vi "Numeric Indicator - Ring.vi"() -> ()   [LabVIEW 2013, in "Ring Workspace Object.lvlib"]
doc: "Sample numeric display item."
uses:
  Ring Workspace Object.lvlib
  <vilib>/NI Veristand/Display Template Support/Display Template Support.llb/cluster_Screen Item Settings.ctl
  <vilib>/NI Veristand/Display Template Support/Display Template Support.llb/cluster_Graph Scale Settings.ctl
  <vilib>/NI Veristand/Display Template Support/Display Template Support.llb/cluster_Graph Plot Settings.ctl
  NationalInstruments.VeriStand.SystemStorage
  <vilib>/NI Veristand/Display Template Support/Display Template Support.llb/enum_Display Template Handler Minimal To Widget Msg.ctl
  <vilib>/NI Veristand/Display Template Support/Display Template Support.llb/enum_Display Template Handler Minimal To Workspace.ctl
  Types/Saved State Data.ctl
  <vilib>/NI Veristand/Display Template Support/Display Template Support.llb/sub_Display Template Handler Custom.vi
  <vilib>/NI Veristand/Execution/Workspace/NI VeriStand - Get Single Channel Value.vi
  <vilib>/NI Veristand/Execution/Workspace/NI_VS Workspace ExecutionAPI.lvlib
panel:
  out "Ring":i64(ring) caption="Channel"
  in  "NIVS.System Definition Root":refnum<k24>
  in  "Item.Data":T1
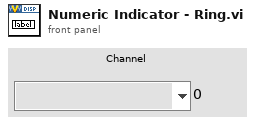
[diagram p1: front panel]
types:
  T1 = typedef "cluster_Screen Item Settings.ctl" = cluster{"Template VI":string, "Position X":i32, "Position Y":i32, "Custom":string, "Show Title Bar":bool, "ID":i32, "Always On Top":bool, "Allow Resize":bool, "Allow Minimize":bool, "Allow Close":bool, "Size to Screen":bool, "Screen.ID":i32, "State":enum16{"Normal", "New"}, "Title":string, "Window Bounds":cluster{"[0]":i16, "[1]":i16, "[2]":i16, "[3]":i16}, "Channel Ref":u64, "Unit":string, "Default Units?":bool, "Flash Limit?":bool, "Color 1":u32, "Color 2":u32, "Color 3":u32, "Color 4":u32, "Bck Color":u32, "Fore Color":u32, "Limit 1":dbl, "Limit 2":dbl, "Limit 3":dbl, "Limit 4":dbl, "Limit Mode 1":i32, "Limit Mode 2":i32, "Limit Mode 3":i32, "Limit Mode 4":i32, "Scale Precision":i32, "Scale Min":dbl, "Scale Max":dbl, "Format":i32, "Precision":i32, "Background Type":i32, "IDs":i32[], "Units":string[], "Labels":string[], "Scale Factor":dbl, "Scale Offset":dbl, "YScale Index":u32[], "XScale":T2, "YScales":T2[], "Plots":T3[], "Update Period":dbl, "History Length":dbl, "My.Ref":refnum<vi>, "Is Control?":bool, "Channel Paths":string[], "Custom Data":variant}
  T2 = typedef "cluster_Graph Scale Settings.ctl" = cluster{"Format":u8, "Precision":u8, "Fit":u8, "Label":string, "Use Default Label":bool, "Label Visible":bool, "Min":dbl, "Max":dbl}
  T3 = typedef "cluster_Graph Plot Settings.ctl" = cluster{"Bar Style":u8, "Fill To":i16, "Fill/PtColor":u32, "Line Style":u8, "Line Width":u8, "Color":u32, "Interp":u8, "Point Style":u8}
  T4 = typedef "enum_Display Template Handler Minimal To Workspace.ctl" = cluster{"Operation":enum16{"SetCustomData", "DeleteItem"}, "Data":variant}
  T5 = typedef "enum_Display Template Handler Minimal To Widget Msg.ctl" = enum16{"Stop", "LaunchConfigDialog"}
  T6 = typedef "Ring Workspace Object.lvlib/Saved State Data.ctl" = cluster{"Name":string, "Node Path":string, "Caption":string, "Value Pairing":string[][]}
  T7 = typedef "NI_VS Workspace ExecutionAPI.lvlib/WorkspaceAPI.ctl" = refnum<k24>
  T8 = typedef "NI_VS UI Single Node Browser.lvlib/Node Ref.ctl" = refnum<k24>
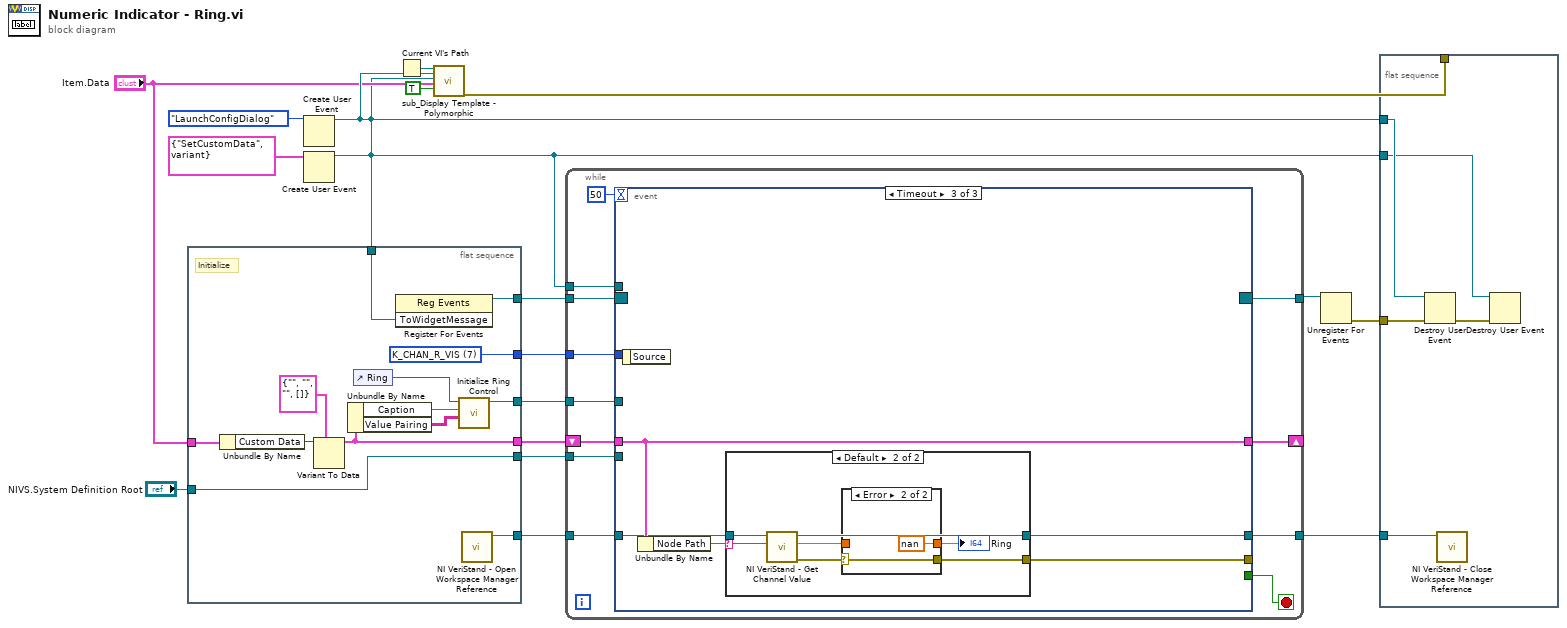
[diagram p0: block diagram]
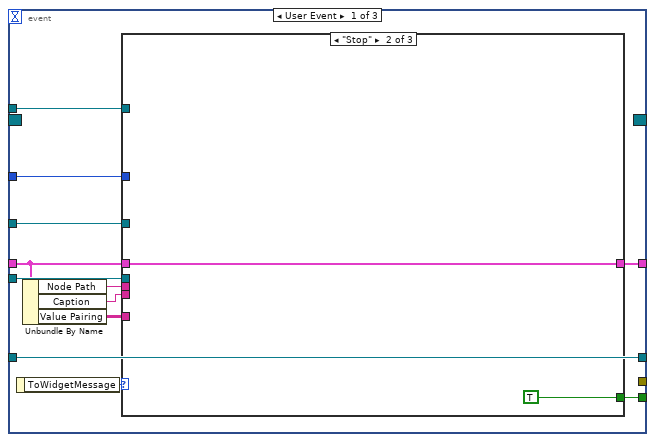
[diagram p2: hidden frame]
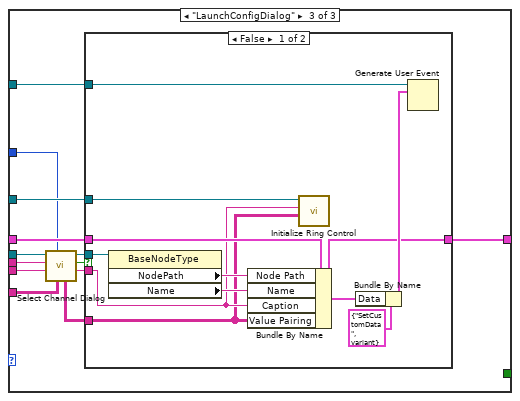
[diagram p4: hidden frame]
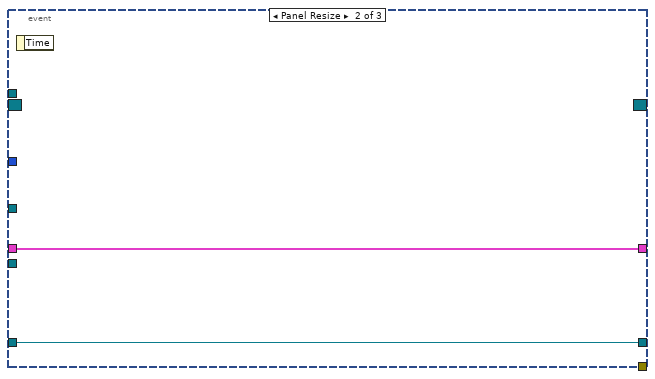
[diagram p6: hidden frame]
diagram:
  n1 = flat-sequence {
    tunnel: [w31] -> w16
    tunnel: w13 -> [w30]
    tunnel: "Item.Data" -> [w29]
    tunnel: [w22] -> w7
    tunnel: "NIVS.System Definition Root" -> [w25]
    tunnel: [w25] -> w5
    tunnel: [w26] -> w4
    tunnel: [w23] -> w3
    tunnel: [w19] -> w1
    frame #0 {
      w19 = u8 7 items=["K_CHAN_R", "K_CHAN_W", "K_CHAN_RW", "K_CHAN_VOLT", "K_CHAN_FAULT", "K_ALL", "K_CUSTOM", "K_CHAN_R_VIS", "K_CHAN_W_VIS", "K_CHAN_RW_VIS", "K_CHAN_VOLT_VIS", "K_CHAN_FAULT_VIS"] ("DisplayFilter")
      # "Initialize"
      n2 = Unbundle By Name(w29) -> ("Custom Data"=w28:variant)
      n3 = Variant To Data(type=T6 {"Name"="", "Node Path"="", "Caption"="", "Value Pairing"=[]}, Variant=w28) -> (data=w22:T6)  [unwired: 1 in, 1 out]
      n4 = Unbundle By Name(w22) -> ("Caption"=w21:string, "Value Pairing"=w20:string[][])
      n5 = control-ref of="Ring"() -> (w24:refnum<vi>)
      n6 = register-events(w30) -> (reference out=w31:refnum<event-registration>)  [unwired: 2 in, 1 out]
      n7 = call "Initialize Ring Control.vi"("Values"=w20, "Caption.Text"=w21, "Ring"=w24) -> ("Ring out"=w23:refnum<vi>)  [unwired: 7 in, 1 out]
      n8 = call <vilib>:"NI VeriStand - Open Workspace Manager Reference.vi"() -> ("WorkspaceManager"=w26:T7)  [unwired: 10 in, 1 out]
    }
  }
  n9 = Create User Event(user event datatype=enum_Display_Template_Handler_Minimal_To_Widget_Msg."LaunchConfigDialog" ("ToWidgetMessage")) -> (user event=w13:refnum<user-event>)  [unwired: 1 in, 1 out]
  n10 = Create User Event(user event datatype=T4 {"Operation"=enum."SetCustomData", "Data"=variant} ("Data")) -> (user event=w9:refnum<user-event>)  [unwired: 1 in, 1 out]
  n11 = Current VI's Path() -> (path=w11:path)
  n12 = call-poly <vilib>:"sub_Display Template - Polymorphic.vi"("Parent.Path"=w11, "ToWidgetEvent"=w13, "ToWorkspace"=w9, "Item.Data"="Item.Data", "Resizable"=TRUE) -> ("error out"=w18:errorcluster)  [unwired: 1 in, 13 out]
  n13 = while {
    tunnel: w16 -> [w43]
    tunnel: [w41] -> w15
    tunnel: w9 -> [w40]
    shift-right: [w37] -> _
    shift-left: w7 -> [w39]
    tunnel: w5 -> [w38]
    tunnel: w4 -> [w35]
    tunnel: w3 -> [w34]
    tunnel: [w33] -> w2
    tunnel: w1 -> [w32]
    stop <- w42 stop-if-true
    n14 = event shown="[2] Timeout" {
      selector: w43 -> [_ _ _]
      dyn-events: [_ _ _] -> w41
      timeout: 50 -> [_ _ _]
      tunnel: [w54 _ _] -> w42
      tunnel: w40 -> [w53 _ _]
      tunnel: w39 -> [w49 w85 w90]
      tunnel: w38 -> [w51 _ _]
      tunnel: [w50 w85 w90] -> w37
      tunnel: w35 -> [w44 w84 w89]
      tunnel: [_ _ w88] -> _
      tunnel: w34 -> [w48 _ _]
      tunnel: [w44 w84 w87] -> w33
      tunnel: w32 -> [w45 _ _]
      event User Event {
        n15 = event-data() -> ("ToWidgetMessage"=w55:T5)  [unwired: 1 out]
        n16 = Unbundle By Name(w49) -> ("Node Path"=w52:string, "Caption"=w47:string, "Value Pairing"=w46:string[][])
        n17 = case shown="\"Stop\"" w55 {
          tunnel: [_ TRUE _] -> w54
          tunnel: w53 -> [_ _ w71]
          tunnel: w52 -> [_ _ w68]
          tunnel: w51 -> [_ _ w67]
          tunnel: [w56 w57 w66] -> w50
          tunnel: w49 -> [w56 w57 w65]
          tunnel: w48 -> [_ _ w64]
          tunnel: w47 -> [_ _ w61]
          tunnel: w46 -> [_ _ w60]
          tunnel: w45 -> [_ _ w59]
          frame Default {
          }
          frame "Stop" {
          }
          frame "LaunchConfigDialog" {
            n18 = call "Select Channel Dialog.vi"("Item Names"=w60, "DisplayFilter"=w59, "Caption"=w61, "nodePath"=w68, "NIVS.System Definition Root"=w67) -> ("Caption out"=w63:string, "Cancel?"=w70:bool, "Selected Item"=w69:T8, "Item Names"=w62:string[][])  [unwired: 2 in, 1 out]
            n19 = case shown="False" w70 {
              tunnel: w71 -> [w82 _]
              tunnel: w69 -> [w79 _]
              tunnel: [w75 w83] -> w66
              tunnel: w65 -> [w76 w83]
              tunnel: w64 -> [w74 _]
              tunnel: w63 -> [w73 _]
              tunnel: w62 -> [w72 _]
              frame False {
                n20 = property class="BaseNodeType"(reference=w79) -> ("NodePath"=w78:string, "Name"=w77:string)  [unwired: 1 in, 2 out]
                n21 = Bundle By Name(cluster=w76, "Node Path"=w78, "Name"=w77, "Caption"=w73, "Value Pairing"=w72) -> (w75:T6)
                n22 = call "Initialize Ring Control.vi"("Values"=w72, "Caption.Text"=w73, "Ring"=w74) -> ()  [unwired: 7 in, 2 out]
                n23 = Bundle By Name(cluster=T4 {"Operation"=enum."SetCustomData", "Data"=variant} ("event data"), "Data"=w75) -> (w80:T4)
                n24 = Generate User Event(user event=w82, event data cluster=w80) -> ()  [unwired: 2 in, 2 out]
              }
              frame True {
              }
            }
          }
        }
      }
      event Panel Resize {
        n25 = event-data() -> ()  [unwired: 2 out]
      }
      event Timeout {
        n26 = event-data() -> ()  [unwired: 2 out]
        n27 = Unbundle By Name(w90) -> ("Node Path"=w86:string)
        n28 = case shown="Default" w86 {
          selector: w86 -> [_ w96]
          tunnel: w89 -> [w91 w98]
          tunnel: [_ w92] -> w88
          tunnel: [w91 w97] -> w87
          frame "" {
          }
          frame Default {
            n29 = call-poly <vilib>:"NI VeriStand - Get Channel Value.vi"("Channel"=w96, "WorkspaceManager in"=w98) -> ("error out"=w93:errorcluster, "Value"=w94:dbl, "WorkspaceManager out"=w97:T7)  [unwired: 7 in]
            n30 = case shown="Error" w93 {
              selector: w93 -> [w99 w101]
              tunnel: [w100 nan ("Value")] -> w95
              tunnel: w94 -> [w100 _]
              tunnel: [w99 w101] -> w92
              frame No Error {
              }
              frame Error {
              }
            }
            "Ring" <- w95
          }
        }
      }
    }
  }
  n31 = Unregister For Events(event registration refnum=w15) -> (error out=w14:errorcluster)  [unwired: 1 in]
  n32 = flat-sequence {
    tunnel: w18 -> [_]
    tunnel: w14 -> [w106]
    tunnel: w13 -> [w107]
    tunnel: w9 -> [w104]
    tunnel: w2 -> [w103]
    frame #0 {
      n33 = Destroy User Event(user event=w107, error in=w106) -> (error out=w105:errorcluster)
      n34 = call <vilib>:"NI VeriStand - Close Workspace Manager Reference.vi"("WorkspaceManager"=w103) -> ()  [unwired: 10 in, 1 out]
      n35 = Destroy User Event(user event=w104, error in=w105) -> ()  [unwired: 1 out]
    }
  }
